vi "State_Machine.vi"(8 "error in (no error)":errorcluster caption="entrée d'erreur (pas d'erreur)", 11 "Wait_CloseFixture en entrée":refnum<class "Operator_Information.lvclass">) -> (0 "error out":errorcluster caption="sortie d'erreur", 2 "Json_String":string, 3 "Wait_CloseFixture en sortie":refnum<class "Operator_Information.lvclass">)   [LabVIEW 2020, in "Library Test.lvlib" / "Operator_Information.lvclass"]
uses:
  Operator_Information.lvclass
  Popup/Class Popup Operator_Validation/Class Popup Operator_Information/Class Popup Operator_Information.lvclass
  C:/Users/ngarcin/OneDrive - Altyor/Standard TB/Suite TB45/Class/Popup/Class Popup Operator_Validation/Class Popup Operator_Validation (Default)/Class Popup Operator_Validation (Virtual).lvclass
  C:/Users/ngarcin/OneDrive - Altyor/Standard TB/Suite TB45/Class/Popup/Class Popup (Main)/Class Popup (Main).lvclass
  Commun VI/TypeDef/Variable Printable.ctl
  Operator_Information.lvclass/Operator_Information.ctl
  JSON API/Variant JSON/Variant to JSON.vi
  JSON API/JSON Value/Get Item by name array.vi
  JSON API/JSON Value/JSON Value.lvclass
  Commun VI/Library Commun.lvlib
  JSON API/Get Polymorphic/JSON GetSet.lvlib
  JSON API/Variant JSON/Variant JSON.lvlib
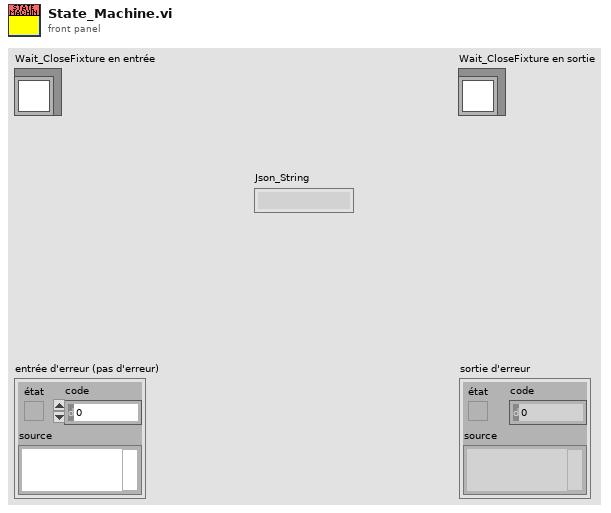
[diagram p1: front panel]
types:
  T1 = enum16{"Get Variable", "Get All Variables", "Set Variable", "Delete Variable", "Delete All Variable"}
  T2 = typedef "Variable Printable.ctl" = string
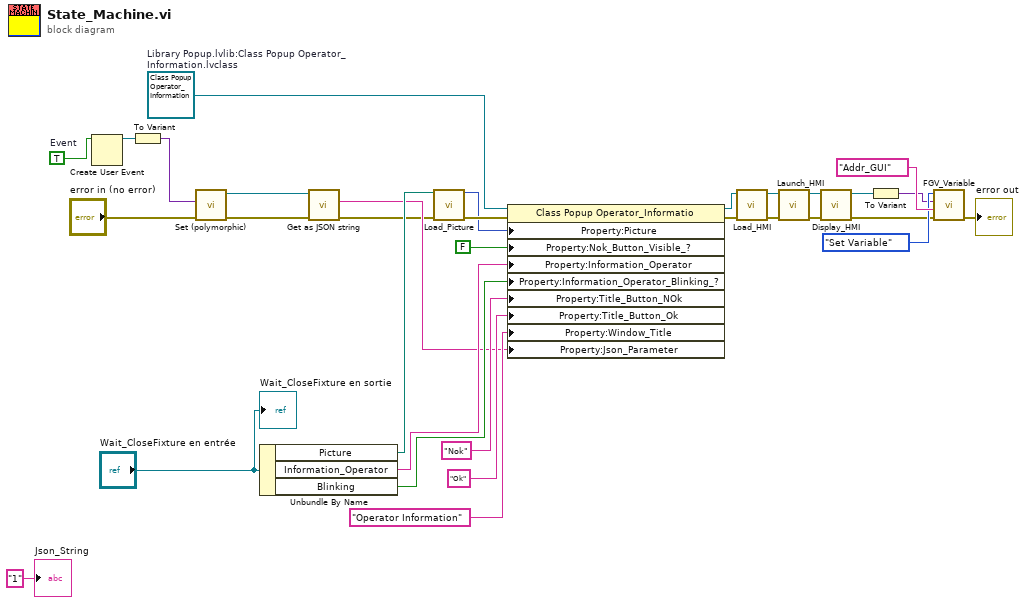
[diagram p0: block diagram]
diagram:
  w14 = TRUE  # Event
  w17 = refnum<class "Class Popup Operator_Information.lvclass"> refnum  # Library Popup.lvlib:Class Popup Operator_Information.lvclass
  n1 = Create User Event(user event datatype=w14) -> (user event=w10:refnum<user-event>)  [unwired: 1 in, 1 out]
  n2 = To Variant(anything=w10) -> (Variant=w13:variant)
  n3 = call-poly "Set (polymorphic).vi"("error in (no error)"="error in (no error)", "Variant"=w13) -> ("error out"=w11:errorcluster, "JSON Value out"=w12:refnum<class "JSON Value.lvclass">)  [unwired: 8 in]
  n4 = Unbundle By Name("Wait_CloseFixture en entrée") -> ("Picture"=w25:path, "Information_Operator"=w28:string, "Blinking"=w27:bool)
  n5 = call "Get as JSON string.vi"("error in (no error)"=w11, "JSON Value in"=w12) -> ("error out"=w7:errorcluster, "<JSON>"=w9:string)  [unwired: 8 in]
  n6 = call "Load_Picture.vi"("Chemin In"=w25, "error in (no error)"=w7) -> ("Img Out"=w24:picture, "error out"=w26:errorcluster)  [unwired: 11 in, 1 out]
  n7 = property class="Class Popup Operator_Informatio"(reference=w17, error in=w26, "Property:Picture"=w24, "Property:Nok_Button_Visible_?"=FALSE ("Nok_Button_Visible_?"), "Property:Information_Operator"=w28, "Property:Information_Operator_Blinking_?"=w27, "Property:Title_Button_NOk"="Nok" ("Title_Button_NOk"), "Property:Title_Button_Ok"="Ok" ("Title_Button_Ok"), "Property:Window_Title"="Operator Information" ("Window_Title"), "Property:Json_Parameter"=w9) -> (reference out=w31:refnum<class "Class Popup Operator_Information.lvclass">, error out=w30:errorcluster)
  n8 = call-dynamic "Load_HMI.vi"("error in (no error)"=w30, "Class Popup (Default) en entrée"=w31) -> ("error out"=w21:errorcluster, "Class Popup (Default) en sortie"=w22:refnum<class "Class Popup Operator_Information.lvclass">)  [unwired: 8 in]
  n9 = call-dynamic "Launch_HMI.vi"("error in (no error)"=w21, "Class Popup (Default) en entrée"=w22) -> ("error out"=w32:errorcluster, "Class Popup (Default) en sortie"=w23:refnum<class "Class Popup Operator_Information.lvclass">)  [unwired: 8 in]
  n10 = call-dynamic "Display_HMI.vi"("error in (no error)"=w32, "Class Popup (Default) en entrée"=w23) -> ("error out"=w4:errorcluster, "Class Popup (Default) en sortie"=w1:refnum<class "Class Popup Operator_Information.lvclass">)  [unwired: 8 in]
  n11 = To Variant(anything=w1) -> (Variant=w2:variant)
  n12 = call "FGV_Variable.vi"("error in (no error)"=w4, "Variable"=T2 "Addr_GUI", "Data In"=w2, "Function"=T1."Set Variable") -> ("error out"=→"error out":errorcluster)  [unwired: 5 in, 2 out]
  "Wait_CloseFixture en sortie" <- "Wait_CloseFixture en entrée"
  "Json_String" <- "1"
